vi "Config Type.vi"(11 "Transition Command in":refnum<class "Transition Command.lvclass">) -> (2 "Command Config Type":refnum<class "Command Config.lvclass">)   [LabVIEW 2020, in "VolatusSeq.lvlib" / "Transition Command.lvclass"]
uses:
  Transition Command.lvclass
  Transition Command.lvclass/Transition Command.ctl
  VolatusSeqConfig/Transition Command Config/Transition Command Config.lvclass
  C:/dev/lv20CE/relink/lv-volatus/VolatusSeqConfig/Command Config/Command Config.lvclass
  C:/dev/lv20CE/relink/lv-volatus/VolatusSeqConfig/Transition Command Config/Transition Command Config.lvclass
  VolatusSeqConfig/Command Config/Command Config.lvclass
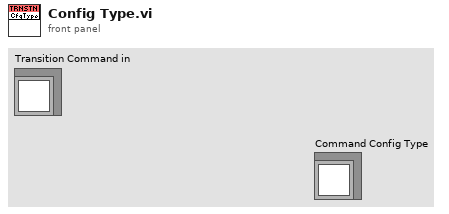
[diagram p1: front panel]
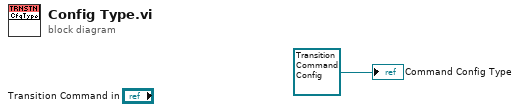
[diagram p0: block diagram]
diagram:
  "Command Config Type" <- refnum<class "Transition Command Config.lvclass"> refnum ("VolatusSeqConfig.lvlib:Transition Command Config.lvclass")
